vi "Client Main.vi"() -> ()   [LabVIEW 2024]
doc: "This VI is the main VI of the client."
uses:
  Controls/Client/Subsystem Overview.ctl
  Controls/Client/Alarm LED.ctl
  Controls/Client/Status LED.ctl
  Controls/Client/Client - Data.ctl
  Support/Shared/Message Queue/Client Message Queues.ctl
  Support/Shared/Message Queue/Message Cluster.ctl
  Controls/Client/Value Change Data.ctl
  Error Handlers/Error Message.ctl
  <vilib>/Utility/cursorutil.llb/Set Cursor (Icon Pict).vi
  Globals/Global - Client.vi
  <vilib>/Utility/cursorutil.llb/Set Cursor (Cursor ID).vi
  Support/Shared/Message Queue.lvlib
  <vilib>/lvdsc/NI_DSC.lvlib
  Support/Shared/User Event - Stop.lvlib
panel:
  out "Server Description":string
  out "Last Archive Time":string
  out "Last Successful Archive Time":string
  out "Next Archive Time":string
  out "Server Running?":T1
  out "Server URL":string
  out "Server Name":string
  out "Subsystem Overview 5":T2
  out "Subsystem Overview 4":T2
  out "Subsystem Overview 3":T2
  out "Subsystem Overview 2":T2
  out "Subsystem Overview 1":T2
  out "Subsystem Overview 0":T2
  in  "Exit":bool
  in  "Open Configuration":bool
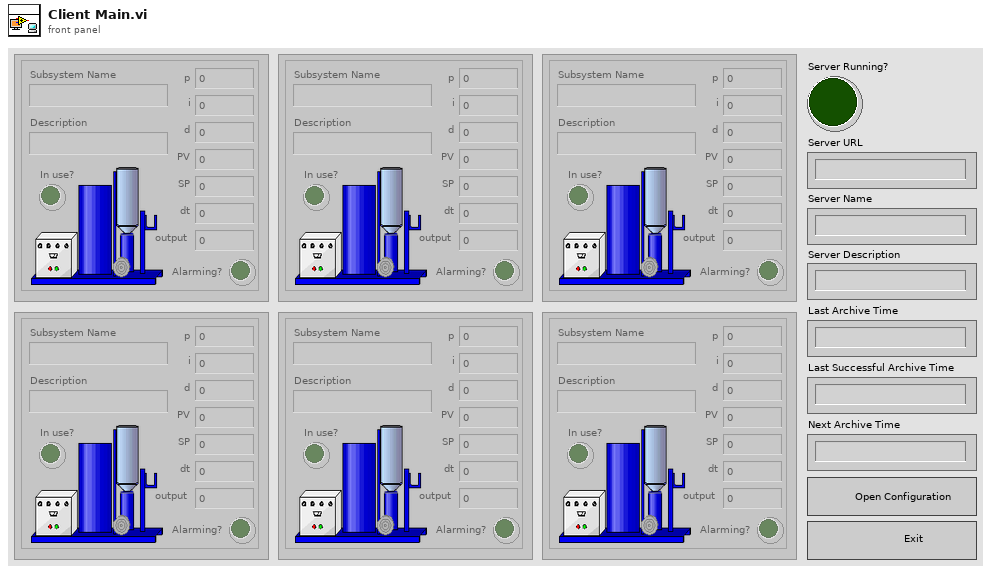
[diagram p1: front panel]
types:
  T1 = typedef "Status LED.ctl" = bool
  T2 = typedef "Subsystem Overview.ctl" = cluster{"Subsystem Name":string, "Description":string, "p":dbl, "i":dbl, "d":dbl, "PV":dbl, "SP":dbl, "dt":dbl, "output":dbl, "Alarming?":T3, "In use?":T1}
  T3 = typedef "Alarm LED.ctl" = bool
  T4 = typedef "Client - Data.ctl" = cluster{"Subsystem Overview Controls":refnum<vi>[], "System Information Controls":refnum<vi>[], "Alarm & Event Notifications":refnum<user-event>, "Value Change Notifications":refnum<user-event>, "Client Message Queues":T5, "Shared Variables":refnum<k21>[], "Subsystem Names":string[], "Server URL":refnum<k21>, "User Event - Stop":refnum<user-event>, "URL Reference Map":variant, "Detailed View VI Reference":refnum<vi>, "Client Configuration File Path":path, "Server Computer":string, "Server Running?":bool}
  T5 = typedef "Message Queue.lvlib/Client Message Queues.ctl" = cluster{"Client Main":refnum<queue>, "Detailed View":refnum<queue>}
  T6 = typedef "Value Change Data.ctl" = cluster{"Shared Variable":refnum<k21>, "Value":variant}
  T7 = enum8{"Enabled", "Disabled", "Disabled and Grayed Out"}
  T8 = typedef "Error Message.ctl" = cluster{"Error":errorcluster, "Component":string}
  T9 = cluster{"Shared Variable":refnum<k21>, "Value":variant}
  T10 = typedef "Client Configuration.ctl" = cluster{"Server URL":refnum<k21>, "Server Computer":string, "Server Name":string}
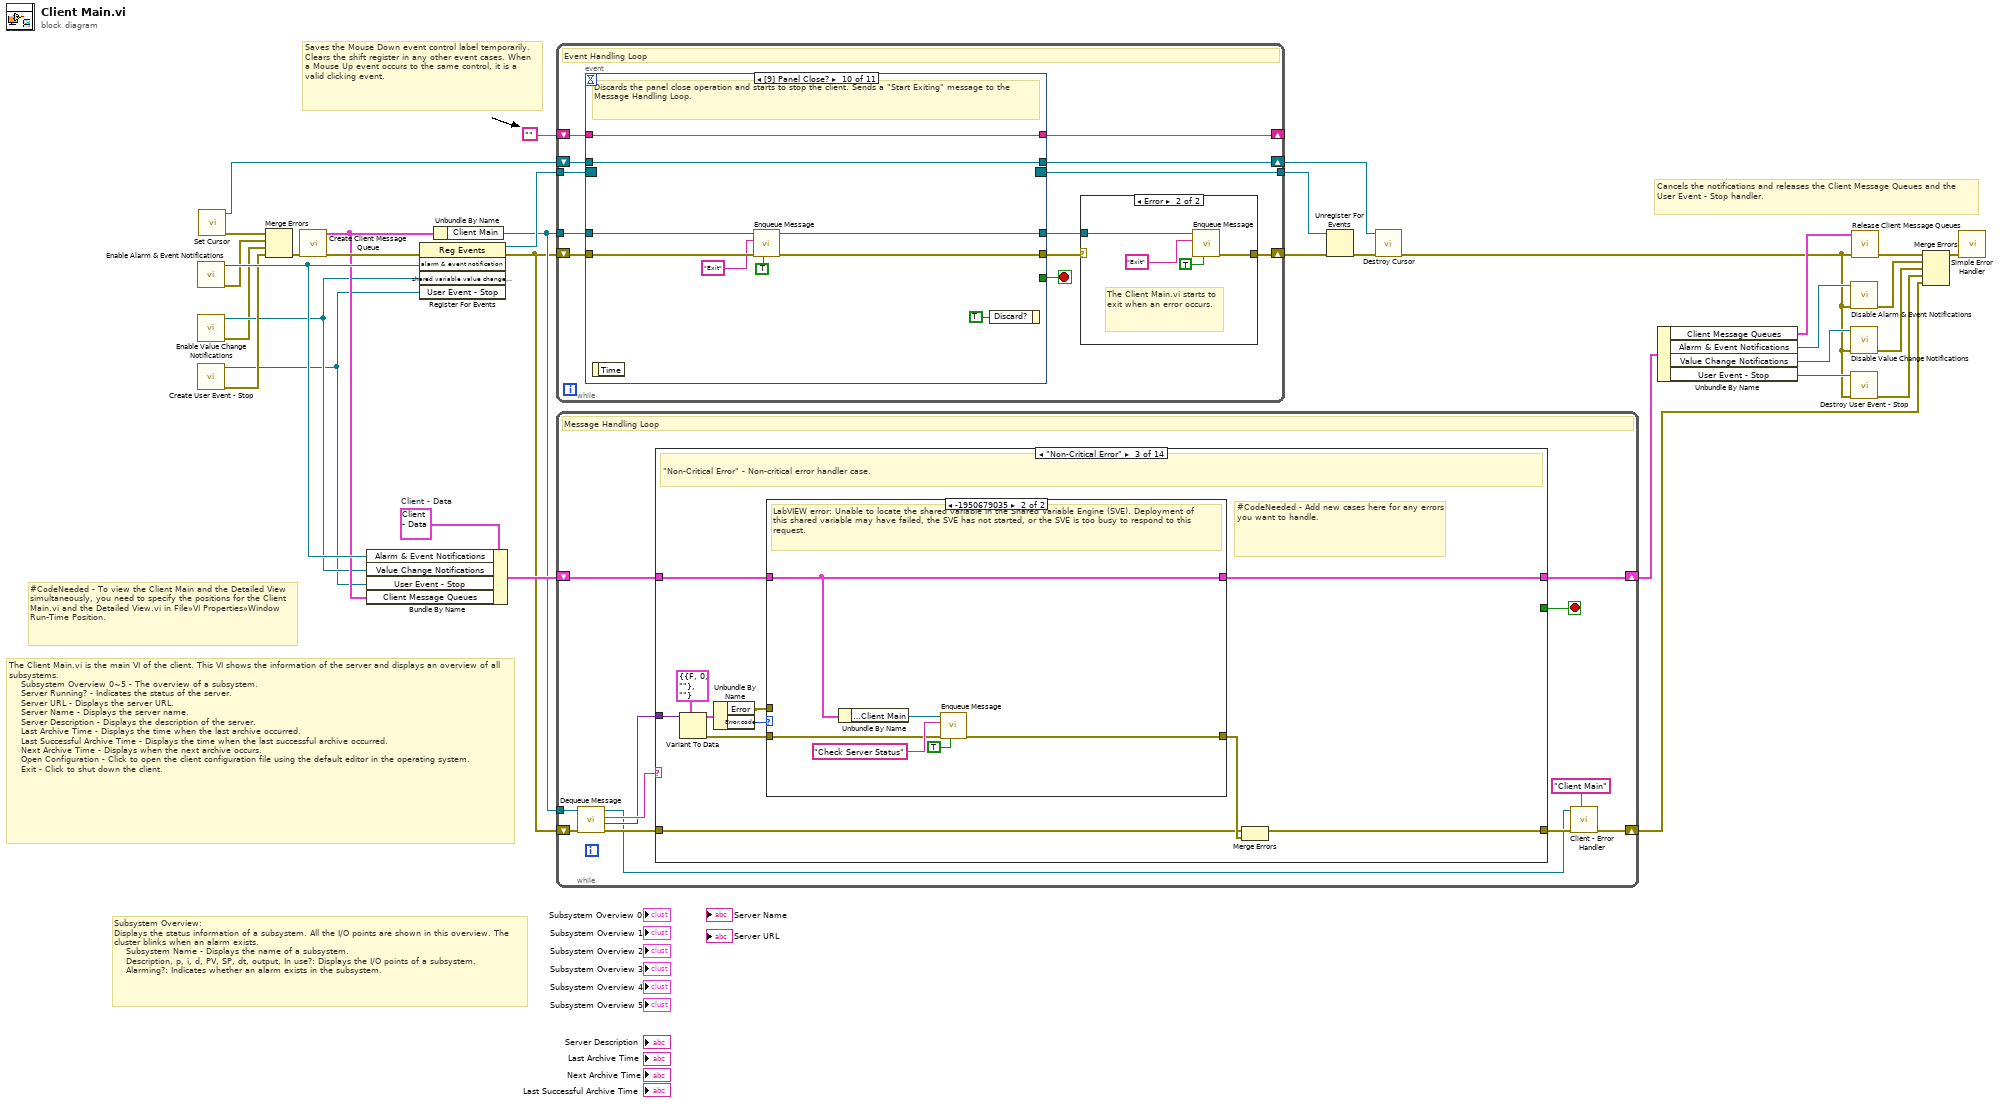
[diagram p0: block diagram]
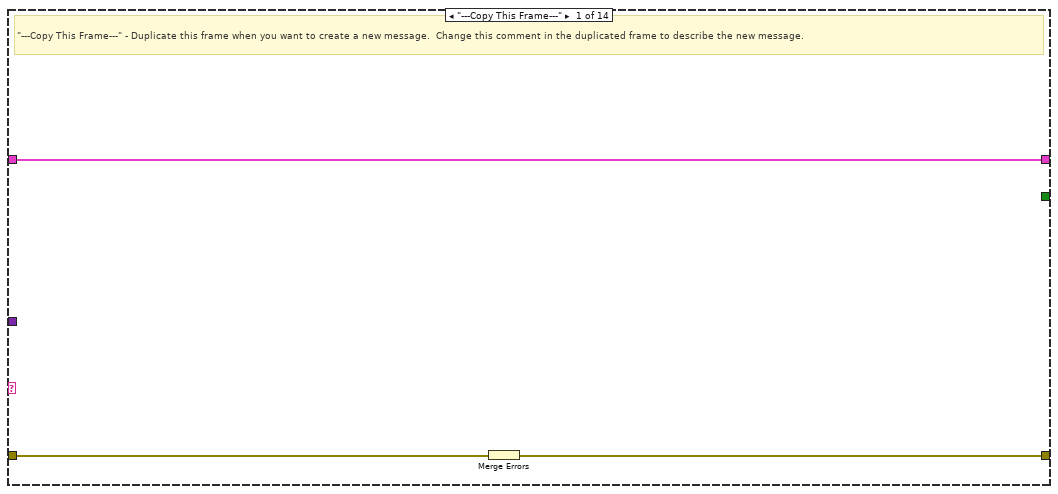
[diagram p2: hidden frame]
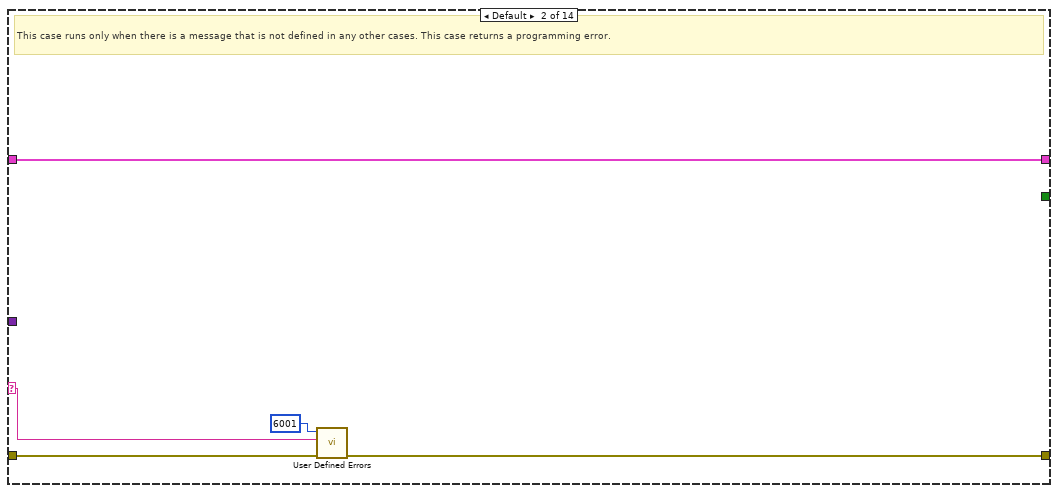
[diagram p3: hidden frame]
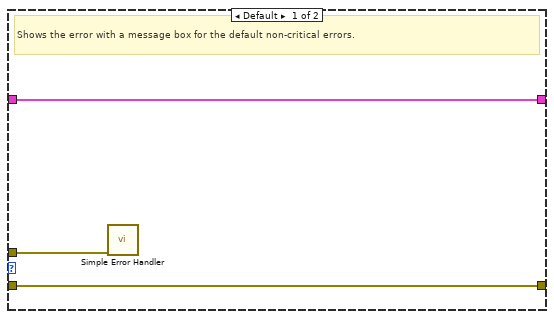
[diagram p4: hidden frame]
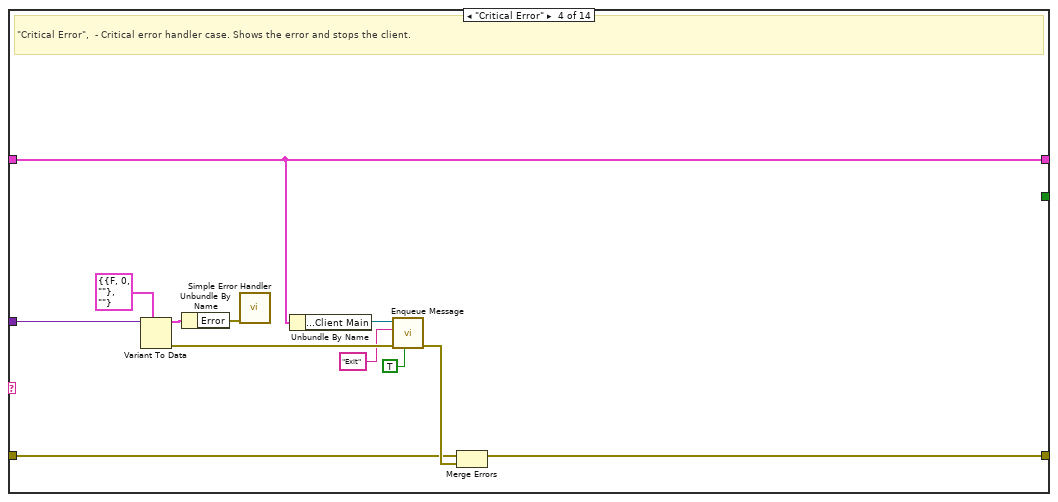
[diagram p5: hidden frame]
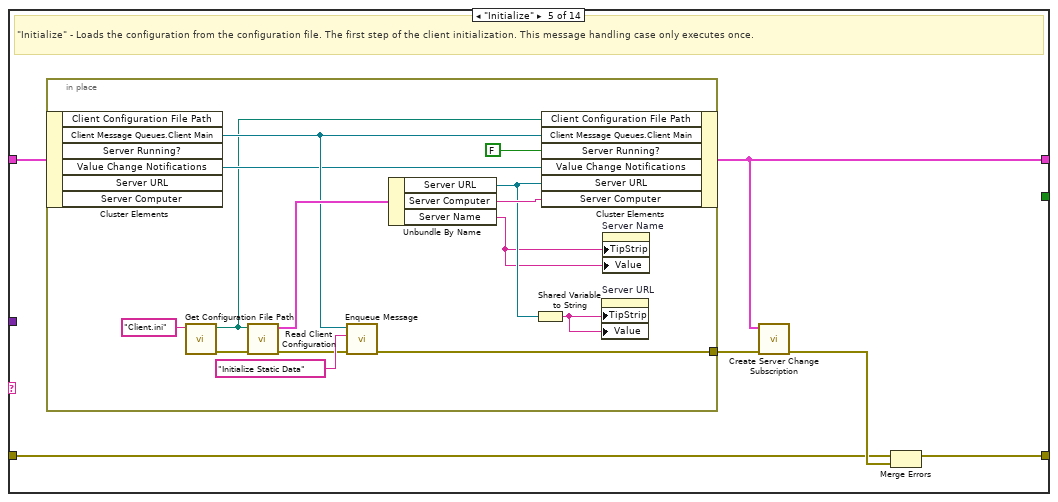
[diagram p6: hidden frame]
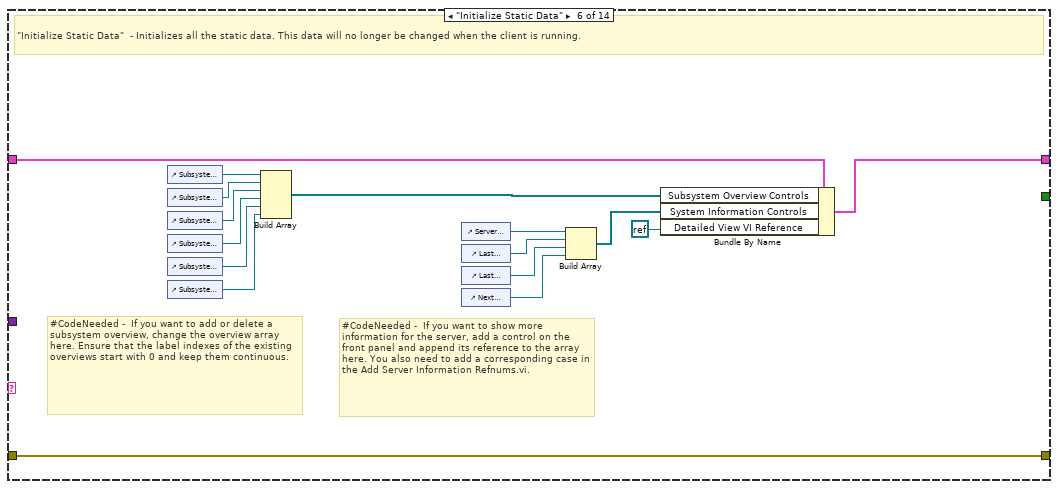
[diagram p7: hidden frame]
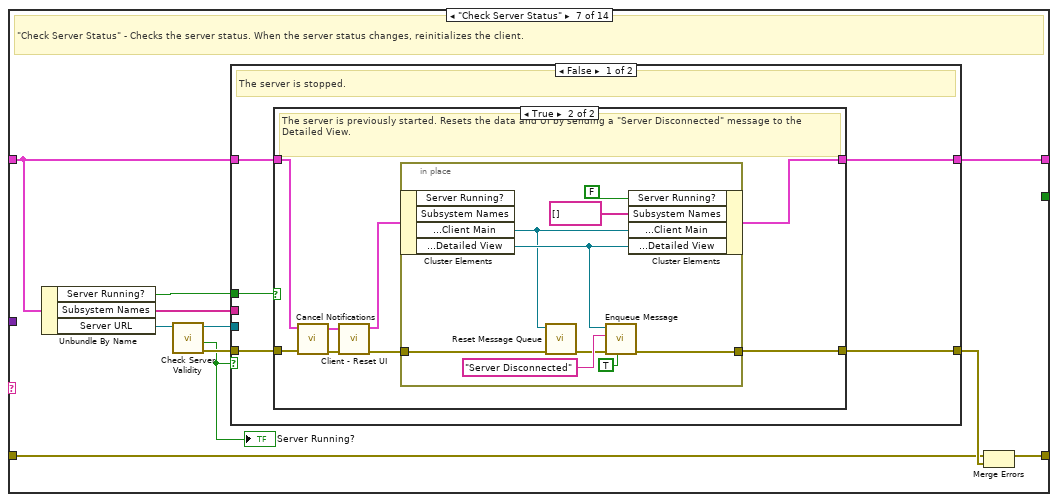
[diagram p8: hidden frame]
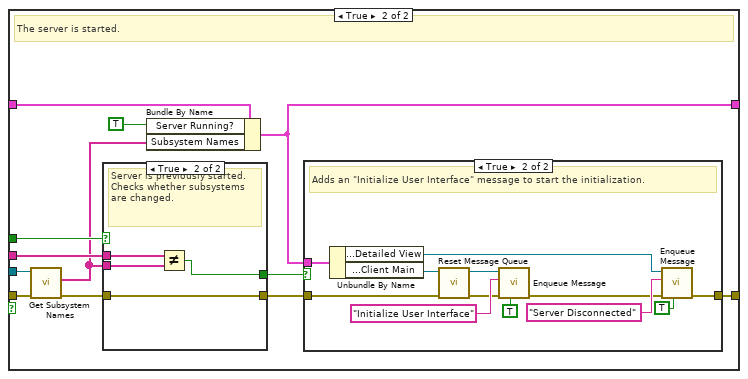
[diagram p10: hidden frame]
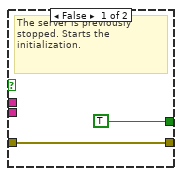
[diagram p12: hidden frame]
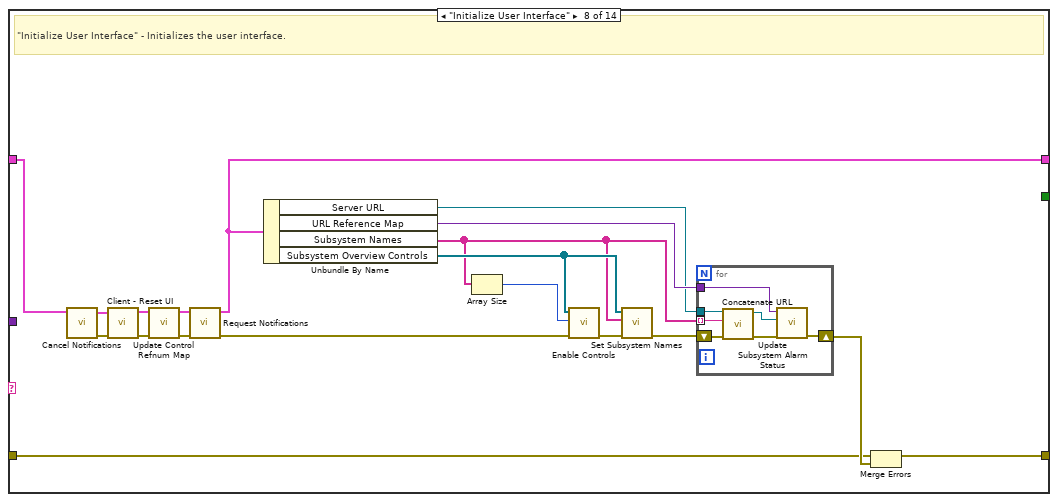
[diagram p13: hidden frame]
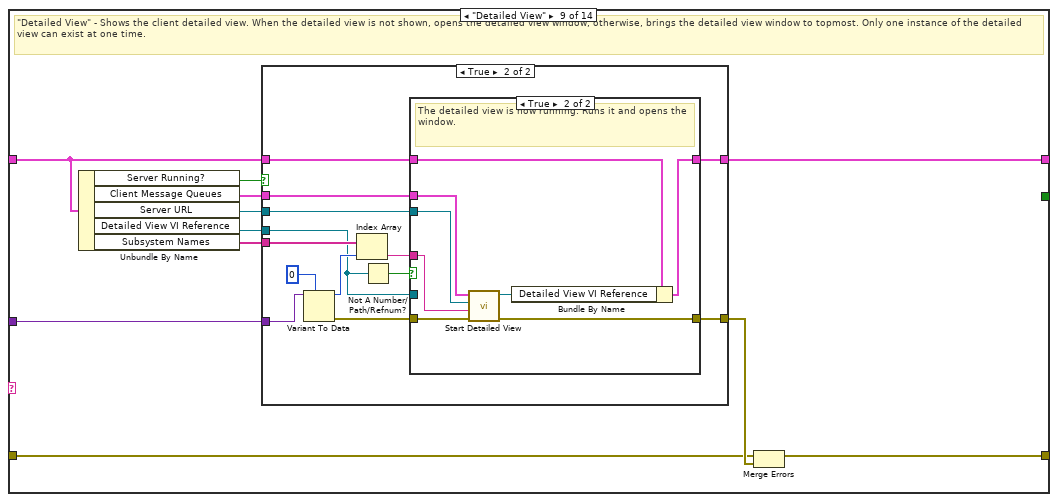
[diagram p14: hidden frame]
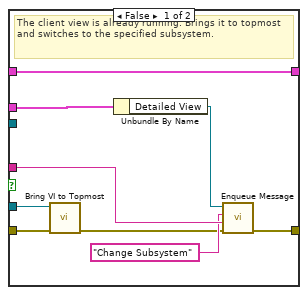
[diagram p16: hidden frame]
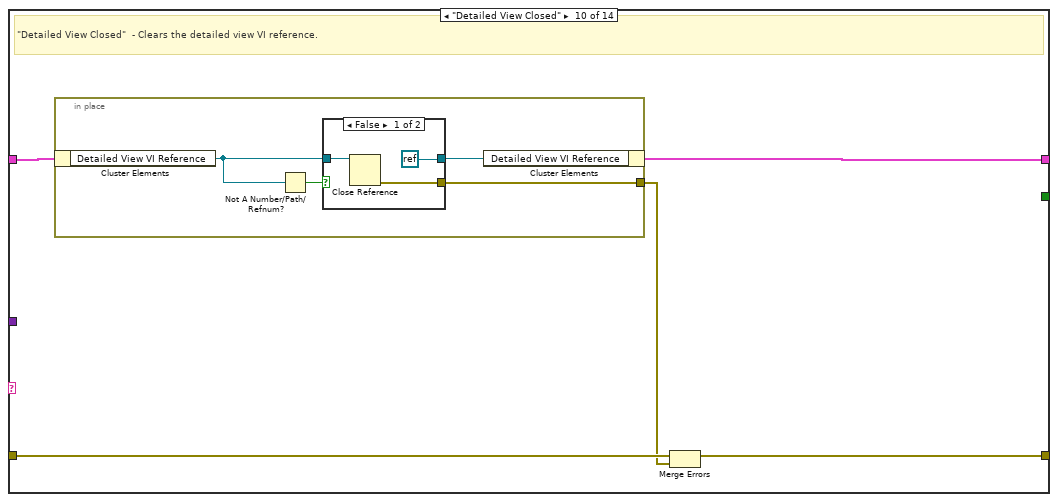
[diagram p17: hidden frame]
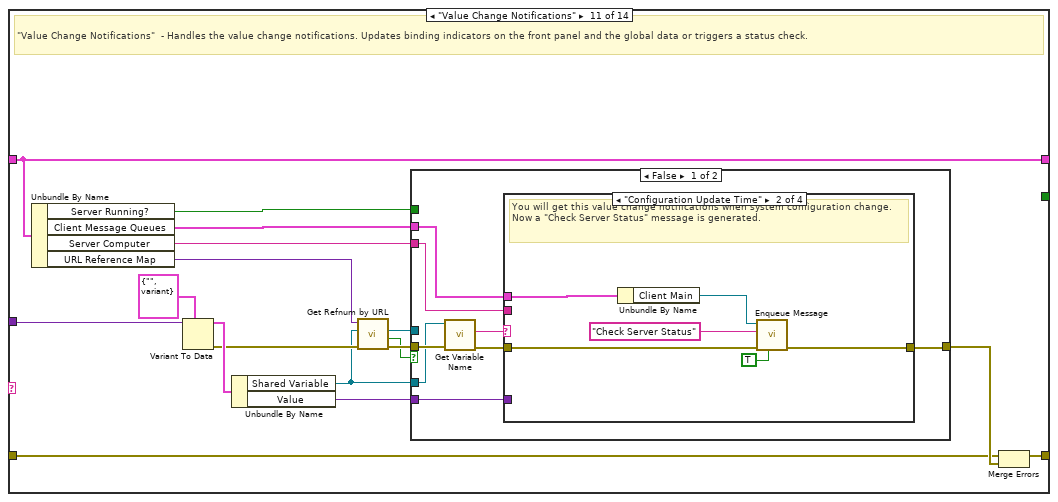
[diagram p19: hidden frame]
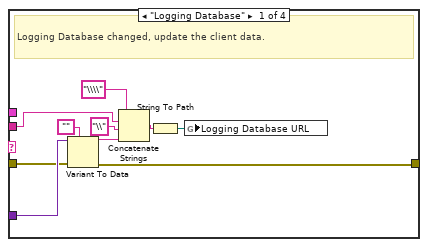
[diagram p20: hidden frame]
diagram:
  w27 = T4 {"Subsystem Overview Controls"=[], "System Information Controls"=[], "Alarm & Event Notifications"=refnum, "Value Change Notifications"=refnum, "Client Message Queues"={"Client Main"=refnum, "Detailed View"=refnum}, "Shared Variables"=[], "Subsystem Names"=[], "Server URL"="", "User Event - Stop"=refnum, "URL Reference Map"=variant, "Detailed View VI Reference"=refnum, "Client Configuration File Path"=path "", "Server Computer"="", "Server Running?"=FALSE}  # Client - Data
  # "#CodeNeeded - To view the Client Main and the Detailed View simultaneously, you need to specify the positions for the Client Main.vi and the Detailed View.vi in File»VI Properties»Window Run-Time Position."
  # "Saves the Mouse Down event control label temporarily. Clears the shift register in any other event cases. When a Mouse Up event occurs to the same control, it is a valid clicking event."
  # "Cancels the notifications and releases the Client Message Queues and the User Event - Stop handler."
  # "The Client Main.vi is the main VI of the client. This VI shows the information of the server and displays an overview of all subsystems.\n    Subsystem Overview 0~5 - The overview of a subsystem.\n    Server Running? - Indicates the status of the server.\n    Server URL - Displays the server URL.\n    Server Name - Displays the server name.\n    Server Description - Displays the description of the server.\n    Last Archive Time - Displays the time when the last archive occurred. \n    Last Successful Archive Time - Displays the time when the last successful archive occurred. \n    Next Archive Time - Displays when the next archive occurs. \n    Open Configuration - Click to open the client configuration file using the default editor in the operating system.\n    Exit - Click to shut down the client."
  # "Subsystem Overview:\nDisplays the status information of a subsystem. All the I/O points are shown in this overview. The cluster blinks when an alarm exists.\n    Subsystem Name - Displays the name of a subsystem.\n    Description, p, i, d, PV, SP, dt, output, In use?: Displays the I/O points of a subsystem.\n    Alarming?: Indicates whether an alarm exists in the subsystem."
  n1 = call <vilib>:"Enable Alarm & Event Notifications.vi"() -> ("error out"=w8:errorcluster, "alarm & event notification"=w33:refnum<user-event>)  [unwired: 10 in]
  n2 = call <vilib>:"Enable Value Change Notifications.vi"() -> ("error out"=w9:errorcluster, "shared variable value change notification"=w10:refnum<user-event>)  [unwired: 10 in]
  n3 = call "Create User Event - Stop.vi"() -> ("error out"=w23:errorcluster, "User Event - Stop"=w1:refnum<user-event>)  [unwired: 10 in]
  n4 = call-poly <vilib>:"Set Cursor.vi"() -> ("error out"=w7:errorcluster, "previous cursor ID"=w6:refnum<k1>)  [unwired: 10 in]
  n5 = Merge Errors(w7, w8, w9, w23) -> (w20:errorcluster)
  n6 = call "Create Client Message Queue.vi"("error in (no error)"=w20) -> ("error out"=w19:errorcluster, "Client Message Queues"=w18:T5)  [unwired: 9 in]
  n7 = Bundle By Name(cluster=w27, "Alarm & Event Notifications"=w33, "Value Change Notifications"=w10, "User Event - Stop"=w1, "Client Message Queues"=w18) -> (w21:T4)
  n8 = register-events(error in=w19, w33, w10, w1) -> (reference out=w32:refnum<event-registration>, error out=w12:errorcluster)  [unwired: 1 in]
  n9 = Unbundle By Name(w18) -> ("Client Main"=w14:refnum<queue>)
  n10 = while "Event Handling Loop" {
    shift-right: [w39] -> w22
    shift-left: w12 -> [w44]
    tunnel: w32 -> [w43]
    tunnel: [w42] -> w31
    tunnel: w14 -> [w41]
    shift-right: [w36] -> w5
    shift-left: w6 -> [w37]
    shift-right: [w34] -> _
    shift-left: "" -> [w35]
    stop <- w45 stop-if-true
    # "Event Handling Loop"
    n11 = event shown="[9] Panel Close?" {
      selector: w43 -> [_ _ _ _ _ _ _ _ _ _ _]
      dyn-events: [_ _ _ _ _ _ _ _ _ _ _] -> w42
      timeout: _ -> [_ _ _ _ _ _ _ _ _ _ _]
      tunnel: [TRUE _ _ _ _ _ _ _ _ _ _] -> w45
      tunnel: w44 -> [w53 w62 w95 w107 w114 w124 w149 w161 w183 w193 w198]
      tunnel: [w53 w61 w92 w106 w113 w122 w148 w164 w182 w191 w197] -> w40
      tunnel: w41 -> [w54 w63 w93 w109 w111 w125 w147 w162 w181 w192 w199]
      tunnel: [w54 w60 w91 w109 w111 w121 w147 w162 w180 w188 w196] -> w38
      tunnel: w37 -> [w52 w57 w90 w108 w115 w127 w142 w166 w179 w186 w195]
      tunnel: [w52 w57 w90 w108 w115 w127 w146 w163 w179 w186 w195] -> w36
      tunnel: w35 -> [w51 w56 w89 w97 _ w120 w140 w159 w178 w185 w194]
      tunnel: [w51 w56 w89 w97 w110 "" ("Label.Text") w140 w159 w178 w185 w194] -> w34
      event User Event {
        # "When the Event Handling Loop receives a user stop event, it stops executing."
        n12 = event-data() -> ()  [unwired: 1 in, 1 out]
      }
      event User Event {
        # "Executes when the quality or value of a registered shared variable changes. Sends a \"Value Change Notifications\" message to the Message Handling Loop."
        n13 = event-data() -> ("Shared Variable"=w64:refnum<k21>, "Value"=w59:variant, "Quality"=w58:u64)  [unwired: 1 in]
        n14 = case shown="0" w58 {
          tunnel: w64 -> [_ w77]
          tunnel: w63 -> [w70 w76]
          tunnel: w62 -> [w68 w75]
          tunnel: [w67 w74] -> w61
          tunnel: [w69 w73] -> w60
          tunnel: w59 -> [_ w72]
          frame Default {
            # "When it's quality change notification, check server status."
            n15 = call "Enqueue Message.vi"("Priority Message? (F)"=TRUE, "error in (no error)"=w68, "Message"="Check Server Status", "Message Queue"=w70) -> ("error out"=w67:errorcluster, "dup Message Queue"=w69:refnum<queue>)  [unwired: 6 in]
          }
          frame 0 {
            n16 = Empty String/Path?(string/path=w72) -> (empty?=w71:bool)
            n17 = case shown="False" w71 {
              tunnel: w77 -> [w84 _]
              tunnel: w72 -> [w83 _]
              tunnel: w76 -> [w82 w87]
              tunnel: w75 -> [w80 w88]
              tunnel: [w79 w88] -> w74
              tunnel: [w78 w87] -> w73
              frame False {
                n18 = Bundle By Name(cluster=T6 {"Shared Variable"="", "Value"=variant} ("Value Change Pair"), "Shared Variable"=w84, "Value"=w83) -> (w81:T6)
                n19 = call "Enqueue Message.vi"("error in (no error)"=w80, "Message Data"=w81, "Message"="Value Change Notifications", "Message Queue"=w82) -> ("error out"=w79:errorcluster, "dup Message Queue"=w78:refnum<queue>)  [unwired: 6 in]
              }
              frame True {
              }
            }
          }
        }
      }
      event User Event {
        # "Executes when the alarm status of a registered shared variable changes. Sends an \"Alarm & Event Notifications\" message to the Message Handling Loop."
        n20 = event-data() -> ("alarm URL"=w94:string)  [unwired: 1 in]
        n21 = call "Enqueue Message.vi"("error in (no error)"=w95, "Message Data"=w94, "Message"="Alarm & Event Notifications", "Message Queue"=w93) -> ("error out"=w92:errorcluster, "dup Message Queue"=w91:refnum<queue>)  [unwired: 6 in]
      }
      event Mouse Down? {
        # "1 stands for left button."
        # "Mouse Down? event. Discards the clicking event when the overview is disabled or the clicking button is not the left mouse button."
        n22 = event-data() -> ("CtlRef"=w105:refnum<vi>, "Button"=w102:u16)  [unwired: 1 in]
        n23 = property class="Clust (strict)"(reference=w105, error in=w107) -> (error out=w106:errorcluster, "DisabledEnum"=w104:T7)  [unwired: 1 out]
        n24 = Not Equal?(x=w104, y=T7."Enabled") -> (x != y?=w100:bool)
        n25 = Not Equal?(x=w102, y=u16 1) -> (x != y?=w99:bool)
        n26 = Or(x=w100, y=w99) -> (x .or. y?=w98:bool)
        n27 = event-data("Discard?"=w98) -> ()  [unwired: 1 in, 1 out]
      }
      event Mouse Down {
        # "Mouse Down event. Saves the control label text to the shift register to help determine whether it is a valid clicking event."
        n28 = event-data() -> ("CtlRef"=w112:refnum<vi>)  [unwired: 1 in]
        n29 = property class="Clust (strict)"(reference=w112, error in=w114) -> (error out=w113:errorcluster, "Label.Text"=w110:string)  [unwired: 1 out]
      }
      event Mouse Up {
        # "Mouse Up event. Opens the Detailed View and shows the corresponding subsystem by sending a \"Detailed View\" message to the Message Handling Loop when a valid clicking event occurs."
        n30 = event-data() -> ("CtlRef"=w123:refnum<vi>)  [unwired: 1 in]
        n31 = property class="Clust (strict)"(reference=w123, error in=w124) -> (error out=w126:errorcluster, "Label.Text"=w117:string)  [unwired: 1 out]
        n32 = Equal?(x=w120, y=w117) -> (x = y?=w119:bool)
        n33 = case shown="True" w119 {
          tunnel: w126 -> [w128 w135]
          tunnel: w125 -> [w129 w134]
          tunnel: [w128 w133] -> w122
          tunnel: [w129 w132] -> w121
          tunnel: "Subsystem Overview" ("string") -> [_ w131]
          tunnel: w117 -> [_ w130]
          frame False {
          }
          frame True {
            n34 = String Length(string=w131) -> (length=w139:i32)
            n35 = String Subset(string=w130, offset (0)=w139) -> (substring=w138:string)  [unwired: 1 in]
            n36 = Octal String To Number(4:w138) -> (0:w136:u32)  [unwired: 2 in, 1 out]
            n37 = call "Enqueue Message.vi"("error in (no error)"=w135, "Message Data"=w136, "Message"="Detailed View", "Message Queue"=w134) -> ("error out"=w133:errorcluster, "dup Message Queue"=w132:refnum<queue>)  [unwired: 6 in]
          }
        }
      }
      event Mouse Enter {
        # "Mouse Enter event. When the cursor enters the overview cluster area, this VI changes the cursor icon to indicate that you can click the overview cluster."
        n38 = event-data() -> ("CtlRef"=w143:refnum<vi>)  [unwired: 1 in]
        n39 = property class="Clust (strict)"(reference=w143, error in=w149) -> (reference out=w144:refnum<vi>, error out=w145:errorcluster, "DisabledEnum"=w141:T7)
        n40 = case shown="\"Enabled\"" w141 {
          tunnel: w145 -> [w156 w158]
          tunnel: [w155 w158] -> w148
          tunnel: [w153 w157] -> w146
          tunnel: w144 -> [w151 _]
          tunnel: w142 -> [_ w157]
          frame "Enabled" {
            # "6 stands for this cursor icon.\nRefer to the LabVIEW Help for more information about other cursor icons."
            n41 = property class="Clust (strict)"(reference=w151, error in=w156, "Color"=u32 11776947) -> (error out=w152:errorcluster)  [unwired: 1 out]
            n42 = call-poly <vilib>:"Set Cursor.vi"("error in (no error)"=w152, "icon"=u16 6) -> ("error out"=w155:errorcluster, "previous cursor ID"=w153:refnum<k1>)  [unwired: 8 in]
          }
          frame Default {
          }
        }
      }
      event Mouse Leave {
        # "Mouse Leave event. Changes the cursor icon to the previous icon when the cursor leaves the overview cluster area."
        n43 = event-data() -> ("CtlRef"=w165:refnum<vi>)  [unwired: 1 in]
        n44 = property class="Clust (strict)"(reference=w165, error in=w161) -> (reference out=w167:refnum<vi>, error out=w168:errorcluster, "DisabledEnum"=w160:T7)
        n45 = case shown="\"Enabled\"" w160 {
          tunnel: w168 -> [w175 w177]
          tunnel: [w174 w177] -> w164
          tunnel: [w173 w176] -> w163
          tunnel: w167 -> [w171 _]
          tunnel: w166 -> [w170 w176]
          frame "Enabled" {
            n46 = property class="Clust (strict)"(reference=w171, error in=w175, "Color"=u32 16777216) -> (error out=w172:errorcluster)  [unwired: 1 out]
            n47 = call-poly <vilib>:"Set Cursor.vi"("error in (no error)"=w172, "cursor ID"=w170) -> ("error out"=w174:errorcluster, "previous cursor ID"=w173:refnum<k1>)  [unwired: 8 in]
          }
          frame Default {
          }
        }
      }
      event "Open Configuration": Value Change {
        # "Opens the configuration file by sending an \"Open Configuration\" message to the Message Handling Loop."
        n48 = event-data() -> ()  [unwired: 1 in, 1 out]
        n49 = call "Enqueue Message.vi"("error in (no error)"=w183, "Message"="Open Configuration", "Message Queue"=w181) -> ("error out"=w182:errorcluster, "dup Message Queue"=w180:refnum<queue>)  [unwired: 7 in]
      }
      event Panel Close? {
        # "Discards the panel close operation and starts to stop the client. Sends a \"Start Exiting\" message to the Message Handling Loop."
        n50 = event-data() -> ()  [unwired: 1 in, 1 out]
        n51 = call "Enqueue Message.vi"("Priority Message? (F)"=TRUE, "error in (no error)"=w193, "Message"="Exit", "Message Queue"=w192) -> ("error out"=w191:errorcluster, "dup Message Queue"=w188:refnum<queue>)  [unwired: 6 in]
        n52 = event-data("Discard?"=TRUE) -> ()  [unwired: 1 in, 1 out]
      }
      event "Exit": Value Change {
        # "Starts to stop the client by sending a \"Start Exiting\" message to the Message Handling Loop."
        n53 = event-data() -> ()  [unwired: 1 in, 1 out]
        n54 = call "Enqueue Message.vi"("Priority Message? (F)"=TRUE, "error in (no error)"=w198, "Message"="Exit", "Message Queue"=w199) -> ("error out"=w197:errorcluster, "dup Message Queue"=w196:refnum<queue>)  [unwired: 6 in]
      }
    }
    n55 = case shown="Error" w40 {
      selector: w40 -> [w46 _]
      tunnel: w38 -> [_ w48]
      tunnel: [w46 w47] -> w39
      frame No Error {
      }
      frame Error {
        # "The Client Main.vi starts to exit when an error occurs."
        n56 = call "Enqueue Message.vi"("Priority Message? (F)"=TRUE, "Message"="Exit", "Message Queue"=w48) -> ("error out"=w47:errorcluster)  [unwired: 7 in, 1 out]
      }
    }
  }
  n57 = while "Message Handling Loop" {
    shift-right: [w204] -> w13
    shift-left: w12 -> [w210]
    shift-right: [w211] -> w17
    shift-left: w21 -> [w212]
    tunnel: w14 -> [w206]
    stop <- w213 stop-if-true
    # "Message Handling Loop"
    n58 = call "Dequeue Message.vi"("error in (no error)"=w210, "Message Queue"=w206) -> ("error out"=w208:errorcluster, "Message Data"=w207:variant, "Message"=w209:string, "dup Message Queue"=w203:refnum<queue>)  [unwired: 6 in]
    n59 = case "Message Cases" shown="\"Non-Critical Error\"" w209 {
      selector: w209 -> [_ w218 _ _ _ _ _ _ _ _ _ _ _ _]
      tunnel: [_ _ _ _ _ _ _ _ _ _ _ _ _ TRUE] -> w213
      tunnel: [w215 w220 w232 w253 w259 w282 w300 w374 w392 w428 w453 w518 w532 w551] -> w205
      tunnel: w212 -> [w216 w219 w224 w244 w258 w283 w298 w360 w388 w426 w448 w515 w531 w537]
      tunnel: [w216 w219 w223 w244 w255 w284 w294 w363 w385 w424 w448 w515 w531 w549] -> w211
      tunnel: w208 -> [w214 w217 w222 w242 w254 w282 w291 w357 w382 w427 w437 w512 w527 w538]
      tunnel: w207 -> [_ _ w229 w249 _ _ _ _ w387 _ w452 w517 _ _]
      frame "---Copy This Frame---" {
        # "\"---Copy This Frame---\" - Duplicate this frame when you want to create a new message.  Change this comment in the duplicated frame to describe the new message."
        n60 = Merge Errors(w214) -> (w215:errorcluster)
      }
      frame Default {
        # "This case runs only when there is a message that is not defined in any other cases. This case returns a programming error."
        n61 = call "User Defined Errors.vi"("error in (no error)"=w217, "Parameter 1"=w218, "Error Code (0)"=6001 ("error code (0)")) -> ("error out"=w220:errorcluster)  [unwired: 8 in]
      }
      frame "Non-Critical Error" {
        # "#CodeNeeded - Add new cases here for any errors you want to handle."
        # "\"Non-Critical Error\" - Non-critical error handler case."
        n62 = Variant To Data(type=T8 {"Error"={"status"=FALSE, "code"=0, "source"=""}, "Component"=""} ("Error Message"), Variant=w229) -> (data=w231:T8, error out=w228:errorcluster)  [unwired: 1 in]
        n63 = Unbundle By Name(w231) -> ("Error"=w225:errorcluster, "Error.code"=w227:i32)
        n64 = case shown="-1950679035" w227 {
          tunnel: w228 -> [w234 w240]
          tunnel: [w234 w239] -> w226
          tunnel: w225 -> [w235 _]
          tunnel: w224 -> [w233 w238]
          tunnel: [w233 w238] -> w223
          frame Default {
            # "Shows the error with a message box for the default non-critical errors."
            n65 = call <vilib>:"Simple Error Handler.vi"("error in (no error)"=w235) -> ()  [unwired: 4 in, 5 out]
          }
          frame -1950679035 {
            # "LabVIEW error: Unable to locate the shared variable in the Shared Variable Engine (SVE). Deployment of this shared variable may have failed, the SVE has not started, or the SVE is too busy to respond to this request."
            n66 = Unbundle By Name(w238) -> ("Client Message Queues.Client Main"=w237:refnum<queue>)
            n67 = call "Enqueue Message.vi"("Priority Message? (F)"=TRUE, "error in (no error)"=w240, "Message"="Check Server Status", "Message Queue"=w237) -> ("error out"=w239:errorcluster)  [unwired: 6 in, 1 out]
          }
        }
        n68 = Merge Errors(w222, w226) -> (w232:errorcluster)
      }
      frame "Critical Error" {
        # "\"Critical Error\",  - Critical error handler case. Shows the error and stops the client."
        n69 = Variant To Data(type=T8 {"Error"={"status"=FALSE, "code"=0, "source"=""}, "Component"=""} ("Error Message"), Variant=w249) -> (data=w252:T8, error out=w251:errorcluster)  [unwired: 1 in]
        n70 = Unbundle By Name(w252) -> ("Error"=w247:errorcluster)
        n71 = call <vilib>:"Simple Error Handler.vi"("error in (no error)"=w247) -> ()  [unwired: 4 in, 5 out]
        n72 = Unbundle By Name(w244) -> ("Client Message Queues.Client Main"=w243:refnum<queue>)
        n73 = call "Enqueue Message.vi"("Priority Message? (F)"=TRUE, "error in (no error)"=w251, "Message"="Exit", "Message Queue"=w243) -> ("error out"=w248:errorcluster)  [unwired: 6 in, 1 out]
        n74 = Merge Errors(w242, w248) -> (w253:errorcluster)
      }
      frame "Initialize" {
        # "\"Initialize\" - Loads the configuration from the configuration file. The first step of the client initialization. This message handling case only executes once."
        n75 = in-place {
          in-place-border: [w266] -> w257
          n76 = in-place-cluster #1(w258) -> ("Client Message Queues.Client Main"=w269:refnum<queue>, "Value Change Notifications"=w267:refnum<user-event>)  [unwired: 4 out]
          n77 = call "Get Configuration File Path.vi"("Configuration File Name"="Client.ini") -> ("error out"=w262:errorcluster, "Configuration File Path"=w260:path)  [unwired: 9 in]
          n78 = call "Read Client Configuration.vi"("error in (no error)"=w262, "Configuration File Path"=w260) -> ("error out"=w268:errorcluster, "Client Configuration"=w272:T10)  [unwired: 8 in]
          n79 = call "Enqueue Message.vi"("error in (no error)"=w268, "Message"="Initialize Static Data", "Message Queue"=w269) -> ("error out"=w266:errorcluster)  [unwired: 7 in, 1 out]
          n80 = Unbundle By Name(w272) -> ("Server URL"=w265:refnum<k21>, "Server Computer"=w270:string, "Server Name"=w264:string)
          n81 = Shared Variable to String(1:w265) -> (0:w263:string)
          n82 = in-place-cluster #1("Client Configuration File Path"=w260, "Client Message Queues.Client Main"=w269, "Server Running?"=FALSE, "Value Change Notifications"=w267, "Server URL"=w265, "Server Computer"=w270) -> (w255:T4)
          n83 = property on="Server URL" class="Str"("TipStrip"=w263, "Value"=w263) -> ()  [unwired: 2 in, 2 out]
          n84 = property on="Server Name" class="Str"("TipStrip"=w264, "Value"=w264) -> ()  [unwired: 2 in, 2 out]
        }
        n85 = call "Create Server Change Subscription.vi"("error in (no error)"=w257, "Client - Data"=w255) -> ("error out"=w256:errorcluster)  [unwired: 8 in, 1 out]
        n86 = Merge Errors(w254, w256) -> (w259:errorcluster)
      }
      frame "Initialize Static Data" {
        # "#CodeNeeded -  If you want to show more information for the server, add a control on the front panel and append its reference to the array here. You also need to add a corresponding case in the Add Server Information Refnums.vi."
        # "#CodeNeeded -  If you want to add or delete a subsystem overview, change the overview array here. Ensure that the label indexes of the existing overviews start with 0 and keep them continuous."
        # "\"Initialize Static Data\"  -\tInitializes all the static data. This data will no longer be changed when the client is running."
        n87 = control-ref of="Subsystem Overview 0"() -> (w279:refnum<vi>)
        n88 = control-ref of="Subsystem Overview 1"() -> (w278:refnum<vi>)
        n89 = control-ref of="Subsystem Overview 2"() -> (w277:refnum<vi>)
        n90 = control-ref of="Subsystem Overview 3"() -> (w276:refnum<vi>)
        n91 = control-ref of="Subsystem Overview 4"() -> (w275:refnum<vi>)
        n92 = control-ref of="Subsystem Overview 5"() -> (w274:refnum<vi>)
        n93 = Build Array(w279, w278, w277, w276, w275, w274) -> (w280:refnum<vi>[])
        n94 = control-ref of="Server Description"() -> (w286:refnum<vi>)
        n95 = control-ref of="Last Archive Time"() -> (w287:refnum<vi>)
        n96 = control-ref of="Last Successful Archive Time"() -> (w288:refnum<vi>)
        n97 = control-ref of="Next Archive Time"() -> (w289:refnum<vi>)
        n98 = Build Array(w286, w287, w288, w289) -> (w285:refnum<vi>[])
        n99 = Bundle By Name(cluster=w283, "Subsystem Overview Controls"=w280, "System Information Controls"=w285, "Detailed View VI Reference"=refnum<k0> refnum) -> (w284:T4)
      }
      frame "Check Server Status" {
        # "\"Check Server Status\" - Checks the server status. When the server status changes, reinitializes the client."
        n100 = Unbundle By Name(w298) -> ("Server Running?"=w299:bool, "Subsystem Names"=w296:string[], "Server URL"=w297:refnum<k21>)
        n101 = call "Check Server Validity.vi"("Server URL"=w297) -> ("error out"=w293:errorcluster, "Valid?"=w292:bool, "dup Server URL"=w290:refnum<k21>)  [unwired: 8 in]
        "Server Running?" <- w292
        n102 = case shown="False" w292 {
          tunnel: w293 -> [w305 w331]
          tunnel: [w303 w332] -> w295
          tunnel: w299 -> [w304 w336]
          tunnel: w298 -> [w302 w327]
          tunnel: [w301 w326] -> w294
          tunnel: w296 -> [_ w335]
          tunnel: w290 -> [_ w329]
          frame False {
            # "The server is stopped."
            n103 = case shown="True" w304 {
              tunnel: w305 -> [w306 w311]
              tunnel: [w306 w308] -> w303
              tunnel: w302 -> [w307 w313]
              tunnel: [w307 w309] -> w301
              frame False {
                # "The server is previously stopped. The status is not changed."
              }
              frame True {
                # "The server is previously started. Resets the data and UI by sending a \"Server Disconnected\" message to the Detailed View."
                n104 = call "Cancel Notifications.vi"("error in (no error)"=w311, "Client - Data In"=w313) -> ("error out"=w314:errorcluster, "Client- Data Out"=w315:T4)  [unwired: 8 in]
                n105 = call "Client - Reset UI.vi"("error in (no error)"=w314, "Client - Data In"=w315) -> ("error out"=w310:errorcluster, "Client - Data Out"=w312:T4)  [unwired: 8 in]
                n106 = in-place {
                  in-place-border: w310 -> [w318]
                  in-place-border: [w320] -> w308
                  n107 = in-place-cluster #2(w312) -> ("Client Message Queues.Client Main"=w316:refnum<queue>, "Client Message Queues.Detailed View"=w319:refnum<queue>)  [unwired: 2 out]
                  n108 = call "Reset Message Queue.vi"("error in (no error)"=w318, "Message Queue"=w316) -> ("error out"=w317:errorcluster)  [unwired: 8 in, 1 out]
                  n109 = call "Enqueue Message.vi"("Priority Message? (F)"=TRUE, "error in (no error)"=w317, "Message"="Server Disconnected", "Message Queue"=w319) -> ("error out"=w320:errorcluster)  [unwired: 6 in, 1 out]
                  n110 = in-place-cluster #2("Server Running?"=FALSE, "Subsystem Names"=string[] [], "Client Message Queues.Client Main"=w316, "Client Message Queues.Detailed View"=w319) -> (w309:T4)
                }
              }
            }
          }
          frame True {
            # "The server is started."
            n111 = call "Get Subsystem Names.vi"("error in (no error)"=w331, "Server URL"=w329) -> ("error out"=w330:errorcluster, "Subsystem Names"=w325:string[])  [unwired: 7 in, 1 out]
            n112 = case shown="True" w336 {
              tunnel: [w350 w352] -> w334
              tunnel: w330 -> [w350 w352]
              tunnel: w335 -> [_ w355]
              tunnel: [TRUE ("Check Server?") w354] -> w333
              tunnel: w325 -> [_ w353]
              frame False {
                # "The server is previously stopped. Starts the initialization."
              }
              frame True {
                # "Server is previously started. Checks whether subsystems are changed."
                n113 = Not Equal?(x=w355, y=w353) -> (x != y?=w354:bool)
              }
            }
            n114 = Bundle By Name(cluster=w327, "Server Running?"=TRUE, "Subsystem Names"=w325) -> (w326:T4)
            n115 = case shown="True" w333 {
              tunnel: w334 -> [w337 w347]
              tunnel: [w337 w344] -> w332
              tunnel: w326 -> [_ w348]
              frame False {
                # "Status is not changed."
              }
              frame True {
                # "Adds an \"Initialize User Interface\" message to start the initialization."
                n116 = Unbundle By Name(w348) -> ("Client Message Queues.Detailed View"=w342:refnum<queue>, "Client Message Queues.Client Main"=w339:refnum<queue>)
                n117 = call "Reset Message Queue.vi"("error in (no error)"=w347, "Message Queue"=w339) -> ("error out"=w340:errorcluster, "dup Message Queue"=w338:refnum<queue>)  [unwired: 8 in]
                n118 = call "Enqueue Message.vi"("Priority Message? (F)"=TRUE, "error in (no error)"=w340, "Message"="Initialize User Interface", "Message Queue"=w338) -> ("error out"=w343:errorcluster)  [unwired: 6 in, 1 out]
                n119 = call "Enqueue Message.vi"("Priority Message? (F)"=TRUE, "error in (no error)"=w343, "Message"="Server Disconnected", "Message Queue"=w342) -> ("error out"=w344:errorcluster)  [unwired: 6 in, 1 out]
              }
            }
          }
        }
        n120 = Merge Errors(w291, w295) -> (w300:errorcluster)
      }
      frame "Initialize User Interface" {
        # "\"Initialize User Interface\" - Initializes the user interface."
        n121 = call "Cancel Notifications.vi"("Client - Data In"=w360) -> ("error out"=w361:errorcluster, "Client- Data Out"=w362:T4)  [unwired: 9 in]
        n122 = call "Client - Reset UI.vi"("error in (no error)"=w361, "Client - Data In"=w362) -> ("error out"=w358:errorcluster, "Client - Data Out"=w359:T4)  [unwired: 8 in]
        n123 = call "Update Control Refnum Map.vi"("error in (no error)"=w358, "Client - Data In"=w359) -> ("error out"=w364:errorcluster, "Client - Data Out"=w365:T4)  [unwired: 8 in]
        n124 = call "Request Notifications.vi"("error in (no error)"=w364, "Client - Data In"=w365) -> ("error out"=w356:errorcluster, "Client - Data Out"=w363:T4)  [unwired: 8 in]
        n125 = Unbundle By Name(w363) -> ("Server URL"=w366:refnum<k21>, "URL Reference Map"=w369:variant, "Subsystem Names"=w372:string[], "Subsystem Overview Controls"=w373:refnum<vi>[])
        n126 = Array Size(array=w372) -> (size(s)=w370:i32)
        n127 = call "Enable Controls.vi"("error in (no error)"=w356, "Number of Enabled Controls"=w370, "Controls"=w373) -> ("error out"=w371:errorcluster)  [unwired: 7 in, 1 out]
        n128 = call "Set Subsystem Names.vi"("error in (no error)"=w371, "Subsystem Names"=w372, "Subsystem Controls"=w373) -> ("error out"=w367:errorcluster)  [unwired: 7 in, 1 out]
        n129 = for {
          tunnel: w366 -> [w380]
          tunnel: w372 -> [w379] mode=indexing
          shift-right: [w377] -> w368
          shift-left: w367 -> [w381]
          tunnel: w369 -> [w376]
          n130 = call "Concatenate URL.vi"("error in (no error)"=w381, "Child Name"=w379, "Parent URL"=w380) -> ("error out"=w378:errorcluster, "Child URL"=w375:refnum<k21>)  [unwired: 7 in]
          n131 = call "Update Subsystem Alarm Status.vi"("error in (no error)"=w378, "Subsystem URL"=w375, "Reference URL Map In"=w376) -> ("error out"=w377:errorcluster)  [unwired: 7 in, 1 out]
        }
        n132 = Merge Errors(w357, w368) -> (w374:errorcluster)
      }
      frame "Detailed View" {
        # "\"Detailed View\" - Shows the client detailed view. When the detailed view is not shown, opens the detailed view window, otherwise, brings the detailed view window to topmost. Only one instance of the detailed view can exist at one time."
        n133 = Unbundle By Name(w388) -> ("Server Running?"=w383:bool, "Client Message Queues"=w386:T5, "Server URL"=w389:refnum<k21>, "Detailed View VI Reference"=w390:refnum<vi>, "Subsystem Names"=w391:string[])
        n134 = case shown="True" w383 {
          tunnel: w391 -> [_ w405]
          tunnel: w390 -> [_ w394]
          tunnel: w389 -> [_ w404]
          tunnel: w388 -> [w393 w403]
          tunnel: w387 -> [_ w402]
          tunnel: w386 -> [_ w399]
          tunnel: [w393 w398] -> w385
          tunnel: [_ w397] -> w384
          frame False {
          }
          frame True {
            n135 = Variant To Data(type=0 ("index"), Variant=w402) -> (data=w400:i32, error out=w396:errorcluster)  [unwired: 1 in]
            n136 = Index Array(array=w405, index=w400) -> (element=w406:string)
            n137 = Not A Number/Path/Refnum?(number/path/refnum=w394) -> (NaN/Path/Refnum?=w395:bool)
            n138 = case shown="True" w395 {
              tunnel: w406 -> [w415 w416]
              tunnel: [w413 w421] -> w397
              tunnel: w396 -> [w412 w420]
              tunnel: w403 -> [w409 w423]
              tunnel: [w409 w422] -> w398
              tunnel: w404 -> [_ w418]
              tunnel: w399 -> [w408 w419]
              tunnel: w394 -> [w407 _]
              frame False {
                # "The client view is already running. Brings it to topmost and switches to the specified subsystem."
                n139 = call "Bring VI to Topmost.vi"("error in (no error)"=w412, "VI Reference In"=w407) -> ("error out"=w411:errorcluster)  [unwired: 8 in, 1 out]
                n140 = Unbundle By Name(w408) -> ("Detailed View"=w410:refnum<queue>)
                n141 = call "Enqueue Message.vi"("error in (no error)"=w411, "Message Data"=w415, "Message"="Change Subsystem", "Message Queue"=w410) -> ("error out"=w413:errorcluster)  [unwired: 6 in, 1 out]
              }
              frame True {
                # "The detailed view is now running. Runs it and opens the window."
                n142 = call "Start Detailed View.vi"("error in (no error)"=w420, "Start Subsystem"=w416, "Server URL"=w418, "Client Message Queues"=w419) -> ("error out"=w421:errorcluster, "VI Reference"=w417:refnum<vi>)  [unwired: 6 in]
                n143 = Bundle By Name(cluster=w423, "Detailed View VI Reference"=w417) -> (w422:T4)
              }
            }
          }
        }
        n144 = Merge Errors(w382, w384) -> (w392:errorcluster)
      }
      frame "Detailed View Closed" {
        # "\"Detailed View Closed\"  - Clears the detailed view VI reference."
        n145 = in-place {
          in-place-border: [w432] -> w425
          n146 = in-place-cluster #3(w426) -> ("Detailed View VI Reference"=w429:refnum<vi>)
          n147 = Not A Number/Path/Refnum?(number/path/refnum=w429) -> (NaN/Path/Refnum?=w430:bool)
          n148 = case shown="False" w430 {
            tunnel: w429 -> [w434 w436]
            tunnel: [w435 _] -> w432
            tunnel: [refnum<k0> refnum w436] -> w431
            frame False {
              n149 = Close Reference(reference=w434) -> (error out=w435:errorcluster)  [unwired: 1 in]
            }
            frame True {
            }
          }
          n150 = in-place-cluster #3("Detailed View VI Reference"=w431) -> (w424:T4)
        }
        n151 = Merge Errors(w427, w425) -> (w428:errorcluster)
      }
      frame "Value Change Notifications" {
        # "\"Value Change Notifications\"  - Handles the value change notifications. Updates binding indicators on the front panel and the global data or triggers a status check."
        n152 = Unbundle By Name(w448) -> ("Server Running?"=w438:bool, "Client Message Queues"=w447:T5, "Server Computer"=w449:string, "URL Reference Map"=w451:variant)
        n153 = Variant To Data(type=T9 {"Shared Variable"="", "Value"=variant} ("Value Change Pair"), Variant=w452) -> (data=w442:T9, error out=w440:errorcluster)  [unwired: 1 in]
        n154 = Unbundle By Name(w442) -> ("Shared Variable"=w439:refnum<k21>, "Value"=w441:variant)
        n155 = call "Get Refnum by URL.vi"("error in (no error)"=w440, "URL"=w439, "Map In"=w451) -> ("error out"=w445:errorcluster, "Found?"=w444:bool, "Control Refnum"=w446:refnum<vi>)  [unwired: 5 in, 1 out]
        n156 = case shown="False" w444 {
          tunnel: w446 -> [_ w493]
          tunnel: w445 -> [w461 w492]
          tunnel: w441 -> [w459 w491]
          tunnel: [w455 w490] -> w450
          tunnel: w449 -> [w458 _]
          tunnel: w439 -> [w457 _]
          tunnel: w447 -> [w454 _]
          tunnel: w438 -> [_ w489]
          frame False {
            n157 = call "Get Variable Name.vi"("error in (no error)"=w461, "Variable URL"=w457) -> ("error out"=w460:errorcluster, "Variable Name"=w456:string)  [unwired: 7 in, 1 out]
            n158 = case shown="\"Configuration Update Time\"" w456 {
              tunnel: w460 -> [w463 w472 w479 w488]
              tunnel: [w462 w474 w478 w488] -> w455
              tunnel: w459 -> [w468 _ w484 _]
              tunnel: w458 -> [w464 _ w480 _]
              tunnel: w454 -> [_ w473 _ _]
              frame "Logging Database" {
                # "Logging Database changed, update the client data."
                n159 = Variant To Data(error in=w463, type="" ("string"), Variant=w468) -> (data=w467:string, error out=w462:errorcluster)
                n160 = Concatenate Strings("\\\\" ("string"), w464, "\\" ("string"), w467) -> (w466:string)
                n161 = String To Path(string=w466) -> (path=w465:path)
                n162 = global write "Global - Client.vi" "Logging Database URL"(w465) -> ()
              }
              frame "Configuration Update Time" {
                # "You will get this value change notifications when system configuration change. Now a \"Check Server Status\" message is generated."
                n163 = Unbundle By Name(w473) -> ("Client Main"=w476:refnum<queue>)
                n164 = call "Enqueue Message.vi"("Priority Message? (F)"=TRUE, "error in (no error)"=w472, "Message"="Check Server Status", "Message Queue"=w476) -> ("error out"=w474:errorcluster)  [unwired: 6 in, 1 out]
              }
              frame "Archive Database" {
                # "Archive Database changed, update the client data."
                n165 = Variant To Data(error in=w479, type="" ("string"), Variant=w484) -> (data=w483:string, error out=w478:errorcluster)
                n166 = Concatenate Strings("\\\\" ("string"), w480, "\\" ("string"), w483) -> (w482:string)
                n167 = String To Path(string=w482) -> (path=w481:path)
                n168 = global write "Global - Client.vi" "Archive Database URL"(w481) -> ()
              }
              frame Default {
                # "Default, do nothing."
              }
            }
          }
          frame True {
            n169 = case shown="True" w489 {
              tunnel: w493 -> [_ w503]
              tunnel: w492 -> [w494 w502]
              tunnel: w491 -> [_ w499]
              tunnel: [w494 w500] -> w490
              frame False {
                # "When Server is not running. Updating front panel control message is not valid. Do nothing."
              }
              frame True {
                # "Code Needed: Add your own case to do special operation on an indicator."
                # "Update the binding indicator"
                n170 = property class="Ctl"(reference=w503, error in=w502, "Value"=w499) -> (reference out=w497:refnum<vi>, error out=w501:errorcluster)
                n171 = property class="Ctl"(reference=w497, error in=w501) -> (reference out=w495:refnum<vi>, error out=w498:errorcluster, "Label.Text"=w496:string)
                n172 = case shown="\"Last Archive Time\", \"Last Successful Archive Time\", \"Next Archive Time\", \"Server Description\"" w496 {
                  tunnel: w498 -> [w504 w511]
                  tunnel: [w504 w510] -> w500
                  tunnel: w499 -> [_ w508]
                  tunnel: w495 -> [_ w505]
                  frame Default {
                  }
                  frame "Last Archive Time", "Last Successful Archive Time", "Next Archive Time", "Server Description" {
                    n173 = Variant To Data(error in=w511, type="", Variant=w508) -> (data=w506:string, error out=w509:errorcluster)
                    n174 = property class="Ctl"(reference=w505, error in=w509, "TipStrip"=w506) -> (error out=w510:errorcluster)  [unwired: 1 out]
                  }
                }
              }
            }
          }
        }
        n175 = Merge Errors(w437, w450) -> (w453:errorcluster)
      }
      frame "Alarm & Event Notifications" {
        # "\"Alarm & Event Notifications\" - Handles alarm and event notifications. Updates binding indicator and blinks when a new unacknowledged alarm occurs."
        n176 = Unbundle By Name(w515) -> ("URL Reference Map"=w514:variant, "Server Running?"=w513:bool)
        n177 = case shown="True" w513 {
          tunnel: w517 -> [_ w526]
          tunnel: [_ w525] -> w516
          tunnel: w514 -> [_ w524]
          frame False {
          }
          frame True {
            n178 = Variant To Data(type="", Variant=w526) -> (data=w522:string, error out=w521:errorcluster)  [unwired: 1 in]
            n179 = call "Get Subsystem from Alarm.vi"("error in (no error)"=w521, "Alarm URL"=w522) -> ("error out"=w520:errorcluster, "Subsystem URL"=w519:refnum<k21>)  [unwired: 8 in]
            n180 = call "Update Subsystem Alarm Status.vi"("error in (no error)"=w520, "Subsystem URL"=w519, "Reference URL Map In"=w524) -> ("error out"=w525:errorcluster)  [unwired: 7 in, 1 out]
          }
        }
        n181 = Merge Errors(w512, w516) -> (w518:errorcluster)
      }
      frame "Open Configuration" {
        # "\"Open Configuration\" - Opens the client configuration file using the default editor of the operating system. Changes in the configuration file do not take effect until the client is restarted."
        n182 = Unbundle By Name(w531) -> ("Client Configuration File Path"=w529:path)
        n183 = flat-sequence {
          tunnel: w529 -> [w533]
          tunnel: [w533] -> w528
          tunnel: [w536] -> w530
          tunnel: w528 -> [w535]
          frame #0 {
            n184 = One Button Dialog(message="Note: Changes in the configuration file do not take effect until the client is restarted.") -> ()  [unwired: 1 in, 1 out]
          }
          frame #1 {
            n185 = call "Open with Default Program.vi"("File Path"=w535) -> ("error out"=w536:errorcluster)  [unwired: 10 in]
          }
        }
        n186 = Merge Errors(w527, w530) -> (w532:errorcluster)
      }
      frame "Exit" {
        # "#CodeNeeded - Clear your own allocated resource."
        # "\"Exit\" - When the Message Handling Loop receives this message, it stops. Clears data and stops the Event Handling Loop by triggering the server stop event."
        n187 = Unbundle By Name(w537) -> ("Client Message Queues.Detailed View"=w550:refnum<queue>, "User Event - Stop"=w547:refnum<user-event>)
        n188 = local write "Server Running?"(FALSE ("Server Running?")) -> ()
        n189 = call "Cancel Notifications.vi"("Clean All?"=TRUE ("Clean all?"), "Client - Data In"=w537) -> ("error out"=w540:errorcluster, "Client- Data Out"=w541:T4)  [unwired: 8 in]
        n190 = call "Client - Reset UI.vi"("error in (no error)"=w540, "Client - Data In"=w541) -> ("error out"=w545:errorcluster, "Client - Data Out"=w549:T4)  [unwired: 8 in]
        n191 = call "Enqueue Message.vi"("Priority Message? (F)"=TRUE, "Message"="Exit", "Message Queue"=w550) -> ("error out"=w546:errorcluster)  [unwired: 7 in, 1 out]
        n192 = call "Fire User Event - Stop.vi"("User Event - Stop"=w547) -> ("error out"=w548:errorcluster)  [unwired: 10 in]
        n193 = Merge Errors(w538, w545, w546, w548) -> (w551:errorcluster)
      }
    }
    n194 = call "Client - Error Handler.vi"("Component"="Client Main", "error in (no error)"=w205, "Message Queue"=w203) -> ("error out"=w204:errorcluster)  [unwired: 8 in]
  }
  n195 = Unregister For Events(event registration refnum=w31, error in=w22) -> (error out=w4:errorcluster)
  n196 = call <vilib>:"Destroy Cursor.vi"("cursor ID"=w5, "error in (no error)"=w4) -> ("error out"=w3:errorcluster)  [unwired: 8 in]
  n197 = Unbundle By Name(w17) -> ("Client Message Queues"=w15:T5, "Alarm & Event Notifications"=w11:refnum<user-event>, "Value Change Notifications"=w26:refnum<user-event>, "User Event - Stop"=w25:refnum<user-event>)
  n198 = call <vilib>:"Disable Alarm & Event Notifications.vi"("error in (no error)"=w3, "notification refnum"=w11) -> ("error out"=w30:errorcluster)  [unwired: 9 in]
  n199 = call <vilib>:"Disable Value Change Notifications.vi"("error in (no error)"=w3, "notification refnum"=w26) -> ("error out"=w29:errorcluster)  [unwired: 9 in]
  n200 = call "Destroy User Event - Stop.vi"("error in (no error)"=w3, "User Event - Stop"=w25) -> ("error out"=w24:errorcluster)  [unwired: 9 in]
  n201 = call "Release Client Message Queues.vi"("error in (no error)"=w3, "Client Message Queues"=w15) -> ("error out"=w16:errorcluster)  [unwired: 9 in]
  n202 = Merge Errors(w16, w30, w29, w24, w13) -> (w28:errorcluster)
  n203 = call <vilib>:"Simple Error Handler.vi"("error in (no error)"=w28) -> ()  [unwired: 4 in, 5 out]
